vi "Winch_MRay.vi"(8 "Setpoints":dbl[](array[numeric]), 9 "Buttons":T1, 10 "Current POT":dbl format="%#_13g", 11 "Winch State":i32) -> (1 "Winch Out":dbl, 3 "Winch State":i32)   [LabVIEW 2013]
uses:
  <vilib>/Rock Robotics/WPI/Joystick/WPI_JoystickButtonState.ctl
panel:
  out "Shoot Ready":bool
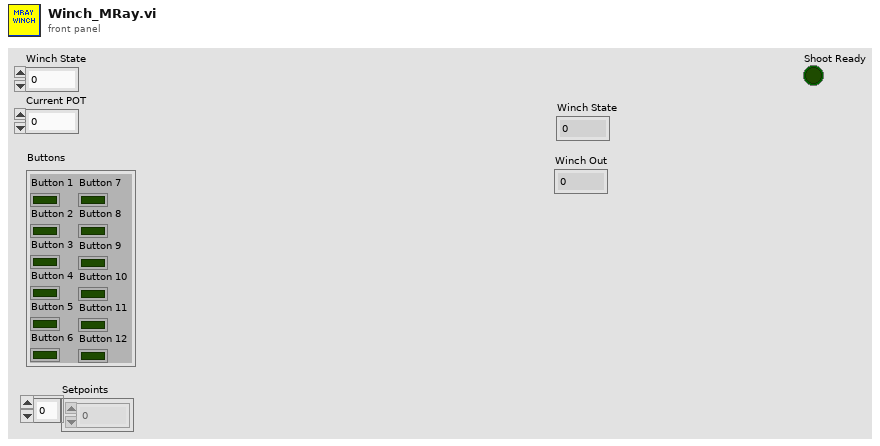
[diagram p1: front panel]
types:
  T1 = typedef "WPI_JoystickButtonState.ctl" = cluster{"Button 1":bool, "Button 2":bool, "Button 3":bool, "Button 4":bool, "Button 5":bool, "Button 6":bool, "Button 7":bool, "Button 8":bool, "Button 9":bool, "Button 10":bool, "Button 11":bool, "Button 12":bool}
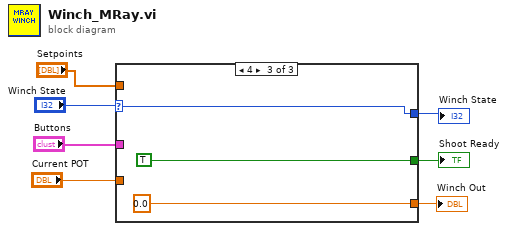
[diagram p0: block diagram]
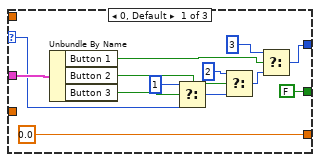
[diagram p2: hidden frame]
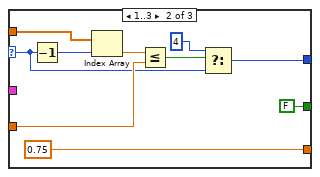
[diagram p3: hidden frame]
diagram:
  n1 = case shown="4" "Winch State" {
    selector: "Winch State" -> [w19 w24 w31]
    tunnel: "Setpoints" -> [_ w29 _]
    tunnel: "Buttons" -> [w20 _ _]
    tunnel: [w10 w23 w31] -> w4
    tunnel: [0.0 ("t") 0.75 ("t") 0.0 ("t")] -> w3
    tunnel: "Current POT" -> [_ w28 _]
    tunnel: [FALSE FALSE TRUE] -> w1
    frame 0, Default {
      n2 = Unbundle By Name(w20) -> ("Button 1"=w13:bool, "Button 2"=w12:bool, "Button 3"=w11:bool)
      n3 = Select(t=1, s=w11, f=w19) -> (s? t:f=w17:i32)
      n4 = Select(t=2, s=w12, f=w17) -> (s? t:f=w15:i32)
      n5 = Select(t=3, s=w13, f=w15) -> (s? t:f=w10:i32)
    }
    frame 1..3 {
      n6 = Decrement(x=w24) -> (x-1=w30:i32)
      n7 = Index Array(array=w29, index=w30) -> (element=w27:dbl)
      n8 = Less Or Equal?(x=w27, y=w28) -> (x <= y?=w26:bool)
      n9 = Select(t=4, s=w26, f=w24) -> (s? t:f=w23:i32)
    }
    frame 4 {
    }
  }
  "Winch State" <- w4
  "Winch Out" <- w3
  "Shoot Ready" <- w1
